vi "Rename_Folder_of_VIs.vi"() -> ()   [LabVIEW 2009]
uses:
  <userlib>/_OpenG.lib/file/file.llb/Build Path - File Names Array__ogtk.vi
  <userlib>/_OpenG.lib/file/file.llb/Strip Path Extension - String__ogtk.vi
  <userlib>/_OpenG.lib/file/file.llb/Strip Path Extension - Path__ogtk.vi
  <userlib>/_OpenG.lib/comparison/comparison.llb/I32 Changed__ogtk.vi
  <userlib>/_OpenG.lib/file/file.llb/Valid Path - Traditional__ogtk.vi
  <userlib>/_OpenG.lib/comparison/comparison.llb/Variant Changed__ogtk.vi
  <userlib>/_OpenG.lib/file/file.llb/Strip Path Extension - 1D Array of Strings__ogtk.vi
panel:
  in  "Swap":bool
  in  "About":bool
  in  "Source Folder":path caption="Folder"
  in  "Folder or LLB":enum32{"Folder", "LLB"}(radio)
  out "Total Progress":u8(slide) scale=0.0..100.0
  out "Progress":u8(slide) scale=0.0..100.0
  in  "Prefix or Suffix":enum32{"Prefix", "Suffix"}(radio)
  in  "Exit Button":bool
  in  "Rename Button":bool
  in  "Recursive":bool
  in  "New Prefix":string caption="New Prefix (\"\": remove existing prefix)"
  in  "Existing Prefix":string caption="Existing Prefix (\"\": prepend new prefix)"
  # "Options"
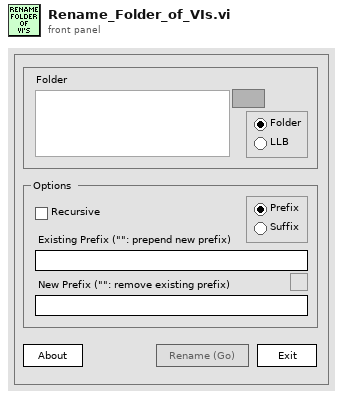
[diagram p1: front panel]
types:
  T1 = cluster{"Version":string, "Build Number":u32, "Build Date/Time":dbl}
  T2 = enum8{"Enabled", "Disabled", "Disabled and Grayed Out"}
  T3 = enum32{"invalid VI type", "Standard VI", "Control VI", "Global VI", "Polymorphic VI", "Configuration VI"}
  T4 = enum32{"invalid VI type", "Standard VI", "Control VI", "Global VI", "Polymorphic VI", "Configuration VI", "SubSystem", "Facade VI", "Method VI", "Statechart Diagram VI"}
  T5 = cluster{"Prompt":string, "Match Pattern":string, "Mode":u32, "Start Path":path}
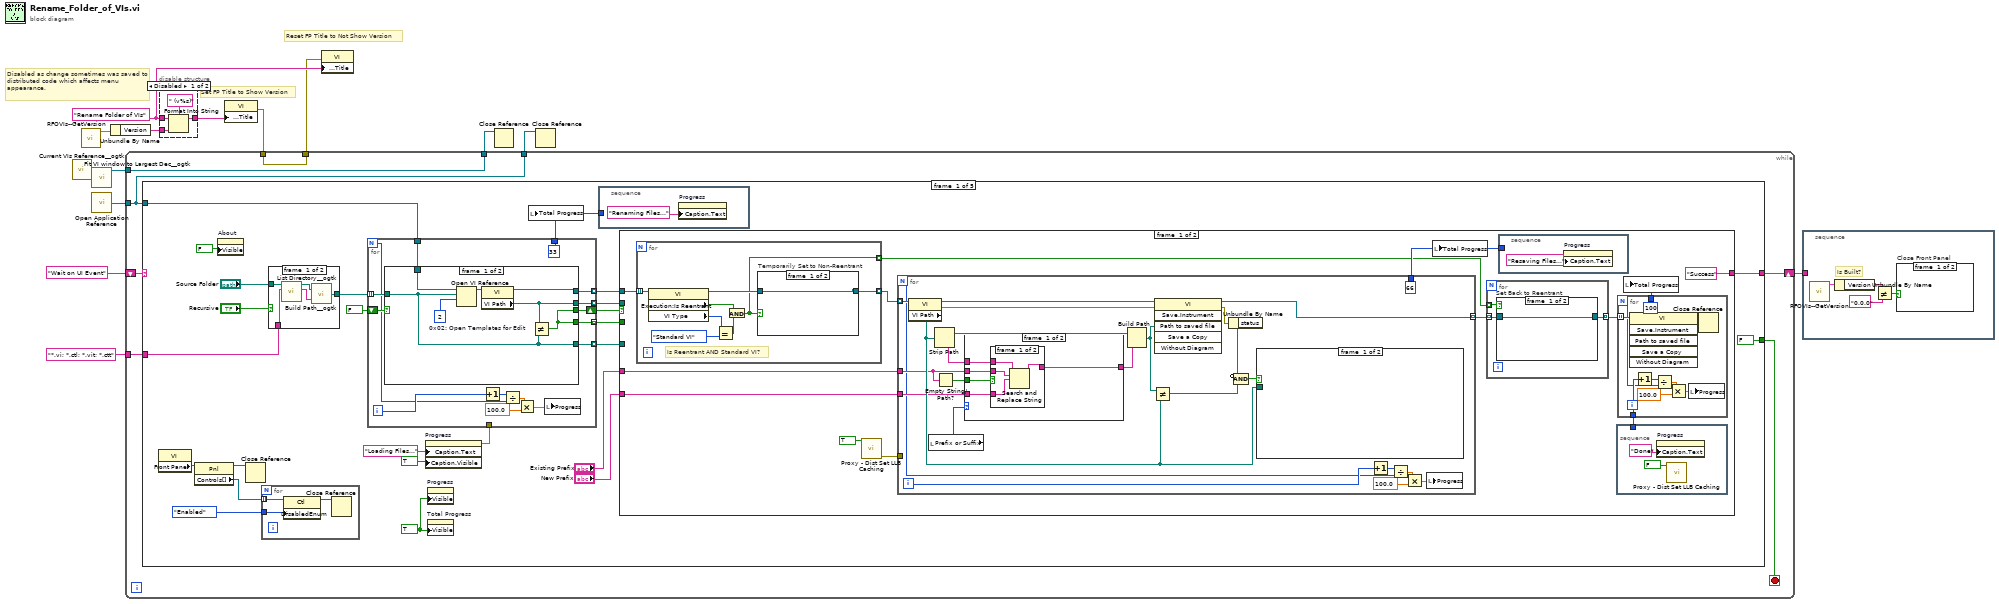
[diagram p0: block diagram]
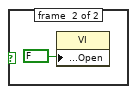
[diagram p3: hidden frame]
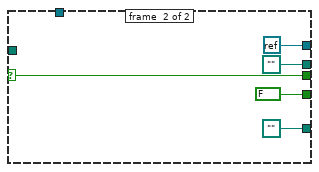
[diagram p4: hidden frame]
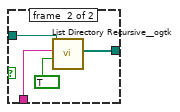
[diagram p5: hidden frame]
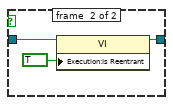
[diagram p6: hidden frame]
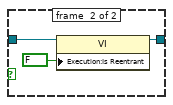
[diagram p7: hidden frame]
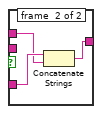
[diagram p8: hidden frame]
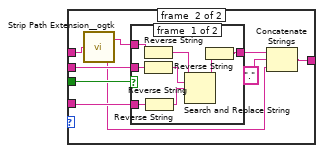
[diagram p9: hidden frame]
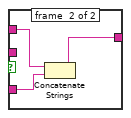
[diagram p10: hidden frame]
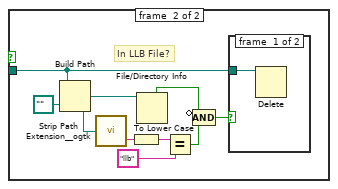
[diagram p11: hidden frame]
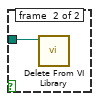
[diagram p12: hidden frame]
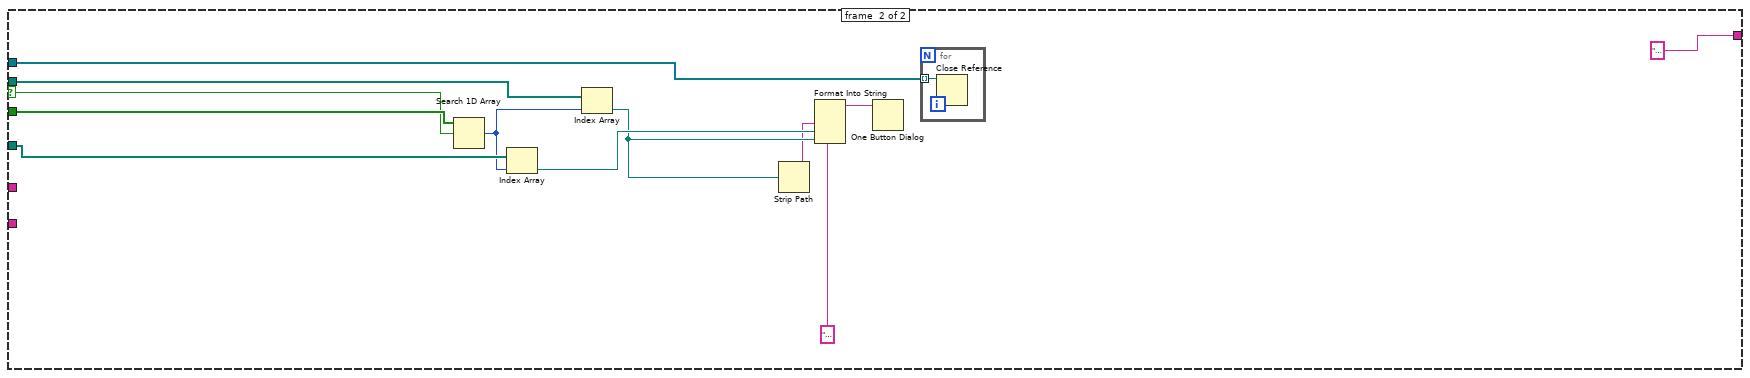
[diagram p13: hidden frame]
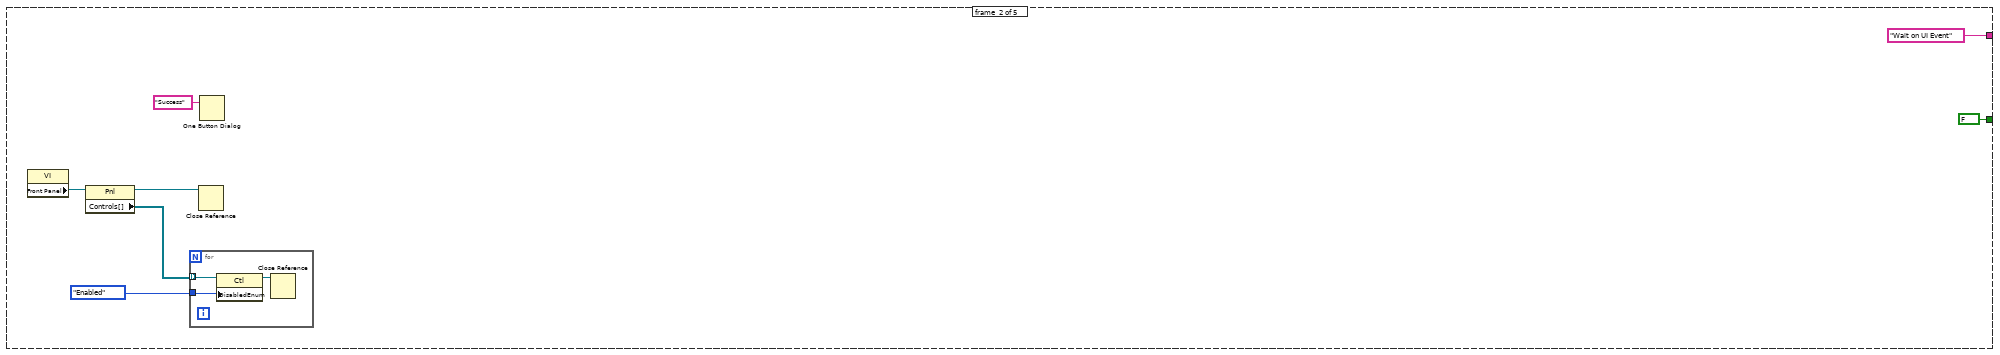
[diagram p14: hidden frame]
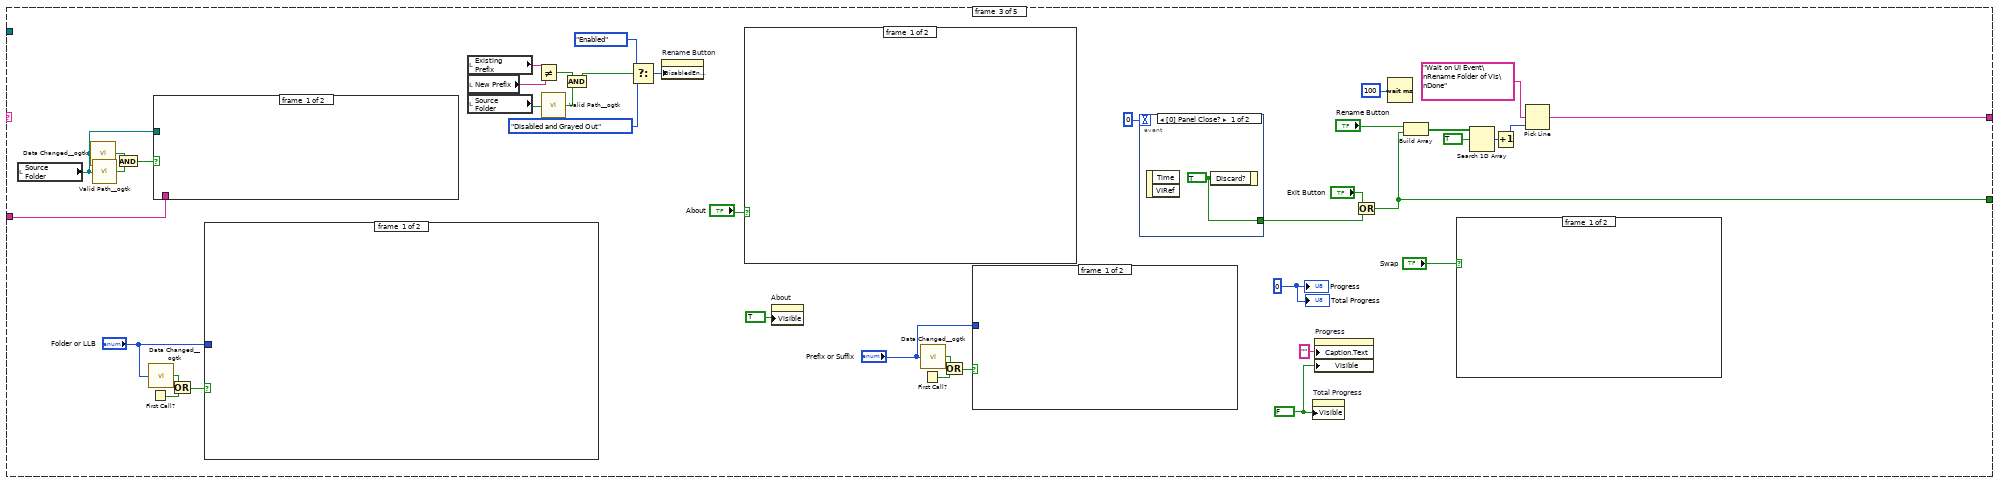
[diagram p15: hidden frame]
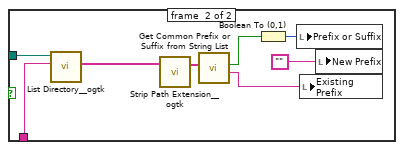
[diagram p16: hidden frame]
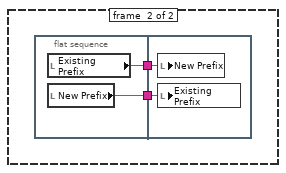
[diagram p17: hidden frame]
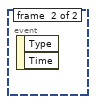
[diagram p18: hidden frame]
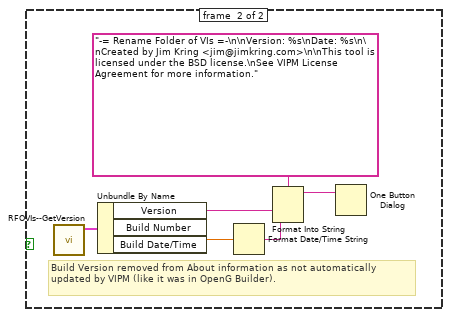
[diagram p19: hidden frame]
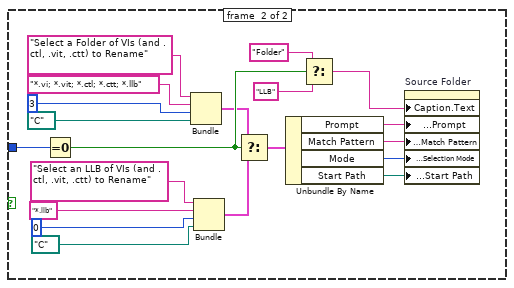
[diagram p20: hidden frame]
diagram:
  w8 = "Rename Folder of VIs" ("format string")
  # "Disabled as change sometimes was saved to distributed code which affects menu appearance."
  # "Set FP Title to Show Version"
  # "Reset FP Title to Not Show Version"
  n1 = call <userlib>:"Current VIs Reference__ogtk.vi"() -> ("Current VI's reference"=w13:refnum<vi>)  [unwired: 5 in]
  n2 = call "RFOVIs--GetVersion.vi"() -> ("Version Info"=w11:T1)  [unwired: 10 in, 1 out]
  n3 = call <userlib>:"Fit VI window to Largest Dec__ogtk.vi"("VI Ref (calling VI)"=w13) -> ("dup VI Ref"=w12:refnum<vi>)  [unwired: 5 in, 1 out]
  n4 = call "Open Application Reference.vi"() -> ("application reference"=w5:refnum<vi>)
  n5 = Unbundle By Name(w11) -> ("Version"=w10:string)
  n6 = disable-structure shown="Disabled" {
    disable-tunnel: w10 -> [w18 _]
    disable-tunnel: [w16 w19] -> w9
    disable-tunnel: w8 -> [w15 w19]
    frame #0 {
      n7 = Format Into String(format string=" (v%s)", initial string=w15, w18) -> (resulting string=w16:string)  [unwired: 1 in, 1 out]
    }
    frame #1 {
    }
  }
  n8 = property class="VI"("Front Panel Window:Title"=w9) -> (error out=w2:errorcluster)  [unwired: 2 in, 1 out]
  n9 = while {
    tunnel: w12 -> [w22]
    shift-left: "Wait on UI Event" -> [w26]
    shift-right: [w24] -> w7
    tunnel: [w23] -> w1
    tunnel: w2 -> [w23]
    tunnel: [w22] -> w6
    tunnel: w5 -> [w21]
    tunnel: [w21] -> w4
    tunnel: "*.vi; *.ctl; *.vit; *.ctt" ("pattern") -> [w20]
    stop <- w25 stop-if-true
    n10 = case shown="\"Wait on UI Event\"" w26 {
      selector: w26 -> [_ _ _ w316 _]
      tunnel: [FALSE ("Cancel") FALSE ("Cancel") w243 FALSE ("Cancel") TRUE ("Cancel")] -> w25
      tunnel: [w27 "Wait on UI Event" ("pattern") w253 "Wait on UI Event" ("pattern") "" ("pattern")] -> w24
      tunnel: w21 -> [w33 _ _ _ _]
      tunnel: w20 -> [w29 _ w230 _ _]
      frame #0 {
        w35 = TRUE ("Visible")
        n11 = property class="VI"() -> ("Front Panel"=w40:refnum<vi>)  [unwired: 2 in, 2 out]
        n12 = property class="Pnl"(reference=w40) -> (reference out=w38:refnum<vi>, "Controls[]"=w39:refnum<vi>[])  [unwired: 1 in, 1 out]
        n13 = property on="About" class="Boolean"("Visible"=FALSE) -> ()  [unwired: 2 in, 2 out]
        n14 = Close Reference(reference=w38) -> ()  [unwired: 1 in, 1 out]
        n15 = for {
          tunnel: w39 -> [w55] mode=indexing
          tunnel: T2."Enabled" ("Disabled") -> [w53]
          n16 = property on="Property Node" class="Ctl"(reference=w55, "DisabledEnum"=w53) -> (reference out=w54:refnum<vi>)  [unwired: 1 in, 1 out]
          n17 = Close Reference(reference=w54) -> ()  [unwired: 1 in, 1 out]
        }
        n18 = case shown="False" "Recursive" {
          tunnel: "Source Folder" -> [w87 w91]
          tunnel: [w83 w90] -> w44
          tunnel: w29 -> [w86 w89]
          frame #0 {
            n19 = call <userlib>:"List Directory__ogtk.vi"("pattern"=w86, "directory path"=w87) -> ("file names"=w84:string[], "dup directory path"=w85:path)  [unwired: 2 in, 2 out]
            n20 = call-poly <userlib>:"Build Path__ogtk.vi"("name or relative path"=w84, "base path"=w85) -> ("appended path"=w83:path[])
          }
          frame #1 {
            n21 = call <userlib>:"List Directory Recursive__ogtk.vi"("Treat llb files as directories? (FALSE)"=TRUE, "pattern"=w89, "Path"=w91) -> ("file paths"=w90:path[])  [unwired: 5 in, 3 out]
          }
        }
        n22 = property on="Progress" class="Slide (strict)"("Caption.Text"="Loading Files...", "Caption.Visible"=TRUE) -> (error out=w31:errorcluster)  [unwired: 2 in, 1 out]
        n23 = for {
          N -> [w58]
          tunnel: w44 -> [w69] mode=indexing
          tunnel: [w70] -> w45 mode=indexing
          shift-right: [w68] -> w48
          shift-left: FALSE -> [w67]
          tunnel: [w66] -> w49 mode=indexing
          tunnel: [w65] -> w50 mode=indexing
          tunnel: [w64] -> w51 mode=indexing
          tunnel: [u8 33 ("Total Progress")] -> w36
          tunnel: w33 -> [w56]
          tunnel: w31 -> [_]
          i -> [w59]
          n24 = case shown="False" w67 {
            selector: w67 -> [_ w82]
            tunnel: [w76 refnum<k0> refnum] -> w70
            tunnel: w69 -> [w73 _]
            tunnel: [w75 w82] -> w68
            tunnel: [w75 FALSE] -> w66
            tunnel: [w73 path ""] -> w65
            tunnel: [w74 path "" ("Path")] -> w64
            tunnel: w56 -> [w71 _]
            frame #0 {
              w72 = 2  # 0x02: Open Templates for Edit
              n25 = Open VI Reference(application reference (local)=w71, vi path=w73, options=w72) -> (vi reference=w77:refnum<vi>)  [unwired: 3 in, 1 out]
              n26 = property class="VI"(reference=w77) -> (reference out=w76:refnum<vi>, "VI Path"=w74:path)  [unwired: 1 in, 1 out]
              n27 = Not Equal?(x=w74, y=w73) -> (x != y?=w75:bool)
            }
            frame #1 {
            }
          }
          n28 = Increment(x=w59) -> (x+1=w60:i32)
          n29 = Divide(x=w60, y=w58) -> (x/y=w62:dbl)
          n30 = Multiply(x=w62, y=100.0) -> (x*y=w63:dbl)
          n31 = local write "Progress"(w63) -> ()
        }
        n32 = property on="Progress" class="Slide (strict)"("Visible"=w35) -> ()  [unwired: 2 in, 2 out]
        n33 = property on="Total Progress" class="Slide (strict)"("Visible"=w35) -> ()  [unwired: 2 in, 2 out]
        n34 = local write "Total Progress"(w36) -> ()
        n35 = stacked-sequence {
          tunnel: w36 -> [_]
          frame #0 {
            n36 = property on="Progress" class="Slide (strict)"("Caption.Text"="Renaming Files...") -> ()  [unwired: 2 in, 2 out]
          }
        }
        n37 = case shown="False" w48 {
          selector: w48 -> [_ w213]
          tunnel: "Existing Prefix" -> [w104 _]
          tunnel: "New Prefix" -> [w103 _]
          tunnel: w45 -> [w98 w212]
          tunnel: w49 -> [_ w214]
          tunnel: w50 -> [_ w211]
          tunnel: w51 -> [_ w210]
          tunnel: ["Success" ("pattern") "Wait on UI Event" ("pattern")] -> w27
          frame #0 {
            n38 = for {
              tunnel: w98 -> [w119] mode=indexing
              tunnel: [w113] -> w94 mode=indexing
              tunnel: [w112] -> w97 mode=indexing
              # "Is Reentrant AND Standard VI?"
              n39 = property class="VI"(reference=w119) -> (reference out=w114:refnum<vi>, "Execution:Is Reentrant"=w115:bool, "VI Type"=w117:T4)  [unwired: 1 in, 1 out]
              n40 = Equal?(x=w117, y=T3."Standard VI" ("VI Type")) -> (x = y?=w116:bool)
              n41 = And(x=w115, y=w116) -> (x .and. y?=w113:bool)
              n42 = case "Temporarily Set to Non-Reentrant" shown="True" w113 {
                tunnel: w114 -> [w120 w123]
                tunnel: [w120 w121] -> w112
                frame #0 {
                }
                frame #1 {
                  n43 = property class="VI"(reference=w123, "Execution:Is Reentrant"=FALSE) -> (reference out=w121:refnum<vi>)  [unwired: 1 in, 1 out]
                }
              }
            }
            n44 = call "Proxy - Dist Set LLB Caching.vi"("enable?"=TRUE) -> ("error out"=w92:errorcluster)  [unwired: 10 in]
            n45 = for {
              N -> [w138]
              tunnel: w104 -> [w149]
              tunnel: w103 -> [w150]
              tunnel: w97 -> [w147] mode=indexing
              tunnel: [w145] -> w96 mode=indexing
              tunnel: [u8 66 ("Total Progress")] -> w101
              tunnel: w92 -> [_]
              i -> [w139]
              n46 = property class="VI"(reference=w147) -> (reference out=w156:refnum<vi>, error out=w155:errorcluster, "VI Path"=w151:path)  [unwired: 1 in]
              n47 = local read "Prefix or Suffix"() -> (w144:enum32{"Prefix", "Suffix"})
              n48 = Strip Path(path=w151) -> (stripped path=w159:path, name=w158:string)
              n49 = Empty String/Path?(string/path=w149) -> (empty?=w148:bool)
              n50 = case shown="\"Prefix\", Default" w144 {
                tunnel: w158 -> [w164 w180]
                tunnel: [w163 w172] -> w157
                tunnel: w150 -> [w162 w177]
                tunnel: w149 -> [w161 w176]
                tunnel: w148 -> [w160 w179]
                frame #0 {
                  n51 = case shown="True" w160 {
                    tunnel: w164 -> [w168 w170]
                    tunnel: [w167 w169] -> w163
                    tunnel: w162 -> [w166 w171]
                    tunnel: w161 -> [w165 _]
                    frame #0 {
                      n52 = Search and Replace String(input string=w168, search string=w165, replace string=w166) -> (result string=w167:string)  [unwired: 5 in, 3 out]
                    }
                    frame #1 {
                      n53 = Concatenate Strings(w171, w170) -> (w169:string)
                    }
                  }
                }
                frame #1 {
                  n54 = call-poly <userlib>:"Strip Path Extension__ogtk.vi"("path"=w180) -> ("root"=w178:string, "extension"=w173:string)
                  n55 = case shown="False" w179 {
                    tunnel: [w184 w191] -> w174
                    tunnel: w177 -> [w187 w189]
                    tunnel: w178 -> [w181 w190]
                    tunnel: w176 -> [w188 _]
                    frame #0 {
                      n56 = Reverse String(1:w181) -> (0:w182:string)
                      n57 = Reverse String(1:w188) -> (0:w186:string)
                      n58 = Reverse String(1:w187) -> (0:w185:string)
                      n59 = Search and Replace String(input string=w182, search string=w186, replace string=w185) -> (result string=w183:string)  [unwired: 5 in, 3 out]
                      n60 = Reverse String(1:w183) -> (0:w184:string)
                    }
                    frame #1 {
                      n61 = Concatenate Strings(w190, w189) -> (w191:string)
                    }
                  }
                  n62 = Concatenate Strings(w174, "." ("Substring"), w173) -> (w172:string)
                }
              }
              n63 = Build Path(base path=w159, name or relative path=w157) -> (appended path=w154:path)
              n64 = Not Equal?(x=w154, y=w151) -> (x != y?=w153:bool)
              n65 = invoke class="VI" method="Save.Instrument"(reference=w156, error in=w155, "Path to saved file"=w154) -> (reference out=w145:refnum<vi>, error out=w146:errorcluster)  [unwired: 3 in, 4 out]
              n66 = Unbundle By Name(w146) -> ("status"=w136:bool)
              n67 = Compound Arithmetic op=AND(invert w136, w153) -> (w152:bool)
              n68 = case shown="True" w152 {
                tunnel: w151 -> [_ w192]
                frame #0 {
                }
                frame #1 {
                  # "In LLB File?"
                  n69 = Build Path(base path=w192, name or relative path=path ".." ("base path")) -> (appended path=w199:path)
                  n70 = call-poly <userlib>:"Strip Path Extension__ogtk.vi"("path"=w199) -> ("extension"=w198:string)  [unwired: 1 out]
                  n71 = To Lower Case(string=w198) -> (all lower case string=w197:string)
                  n72 = File/Directory Info(path=w199) -> (directory=w195:bool)  [unwired: 1 in, 6 out]
                  n73 = Equal?(x=w197, y="llb" ("all lower case string")) -> (x = y?=w194:bool)
                  n74 = Compound Arithmetic op=AND(invert w195, w194) -> (w193:bool)
                  n75 = case shown="True" w193 {
                    tunnel: w192 -> [w201 w202]
                    frame #0 {
                      n76 = Delete(path (use dialog)=w201) -> ()  [unwired: 4 in, 3 out]
                    }
                    frame #1 {
                      n77 = call <vilib>:"Delete From VI Library.vi"("path"=w202) -> ()  [unwired: 10 in, 1 out]
                    }
                  }
                }
              }
              n78 = Increment(x=w139) -> (x+1=w140:i32)
              n79 = Divide(x=w140, y=w138) -> (x/y=w142:dbl)
              n80 = Multiply(x=w142, y=100.0) -> (x*y=w143:dbl)
              n81 = local write "Progress"(w143) -> ()
            }
            n82 = local write "Total Progress"(w101) -> ()
            n83 = for {
              tunnel: [w107] -> w95 mode=indexing
              tunnel: w96 -> [w106] mode=indexing
              tunnel: w94 -> [w105] mode=indexing
              n84 = case "Set Back to Reentrant" shown="True" w105 {
                tunnel: w106 -> [w108 w111]
                tunnel: [w108 w109] -> w107
                frame #0 {
                }
                frame #1 {
                  n85 = property class="VI"(reference=w111, "Execution:Is Reentrant"=TRUE) -> (reference out=w109:refnum<vi>)  [unwired: 1 in, 1 out]
                }
              }
            }
            n86 = stacked-sequence {
              tunnel: w101 -> [_]
              frame #0 {
                n87 = property on="Progress" class="Slide (strict)"("Caption.Text"="Resaving Files...") -> ()  [unwired: 2 in, 2 out]
              }
            }
            n88 = for {
              N -> [w128]
              tunnel: w95 -> [w135] mode=indexing
              tunnel: [u8 100 ("Total Progress")] -> w100
              tunnel: [w129] -> w99
              i -> [w129]
              n89 = invoke class="VI" method="Save.Instrument"(reference=w135) -> (reference out=w134:refnum<vi>)  [unwired: 5 in, 5 out]
              n90 = Increment(x=w129) -> (x+1=w130:i32)
              n91 = Divide(x=w130, y=w128) -> (x/y=w132:dbl)
              n92 = Multiply(x=w132, y=100.0) -> (x*y=w133:dbl)
              n93 = local write "Progress"(w133) -> ()
              n94 = Close Reference(reference=w134) -> ()  [unwired: 1 in, 1 out]
            }
            n95 = stacked-sequence {
              tunnel: w99 -> [_]
              frame #0 {
                n96 = property on="Progress" class="Slide (strict)"("Caption.Text"="Done") -> ()  [unwired: 2 in, 2 out]
                n97 = call "Proxy - Dist Set LLB Caching.vi"("enable?"=FALSE) -> ()  [unwired: 10 in, 1 out]
              }
            }
            n98 = local write "Total Progress"(w100) -> ()
          }
          frame #1 {
            n99 = Search 1D Array(1D array=w214, element=w213) -> (index of element=w209:i32)  [unwired: 1 in]
            n100 = Index Array(array=w211, index=w209) -> (element=w208:path)
            n101 = Index Array(array=w210, index=w209) -> (element=w207:path)
            n102 = Strip Path(path=w207) -> (name=w206:string)  [unwired: 1 out]
            n103 = Format Into String(format string="Cannot rename folder. \"%s\" expected in the following location:\n\n%s\n\nfound already in memory at:\n\n%s\n\nNo VIs renamed.", w206, w208, w207) -> (resulting string=w205:string)  [unwired: 2 in, 1 out]
            n104 = One Button Dialog(message=w205) -> ()  [unwired: 1 in, 1 out]
            n105 = for {
              tunnel: w212 -> [w215] mode=indexing
              n106 = Close Reference(reference=w215) -> ()  [unwired: 1 in, 1 out]
            }
          }
        }
      }
      frame #1 {
        n107 = property class="VI"() -> ("Front Panel"=w220:refnum<vi>)  [unwired: 2 in, 2 out]
        n108 = property class="Pnl"(reference=w220) -> (reference out=w218:refnum<vi>, "Controls[]"=w219:refnum<vi>[])  [unwired: 1 in, 1 out]
        n109 = for {
          tunnel: w219 -> [w225] mode=indexing
          tunnel: T2."Enabled" ("Disabled") -> [w223]
          n110 = property on="Property Node" class="Ctl"(reference=w225, "DisabledEnum"=w223) -> (reference out=w224:refnum<vi>)  [unwired: 1 in, 1 out]
          n111 = Close Reference(reference=w224) -> ()  [unwired: 1 in, 1 out]
        }
        n112 = Close Reference(reference=w218) -> ()  [unwired: 1 in, 1 out]
        n113 = One Button Dialog(message="Success") -> ()  [unwired: 1 in, 1 out]
      }
      frame #2 {
        w251 = FALSE ("Visible")
        w252 = u8 0 ("Progress")
        n114 = local read "Source Folder"() -> (w229:path)
        n115 = call-poly <userlib>:"Data Changed__ogtk.vi"("Variant"=w229) -> ("Changed"=w233:bool)
        n116 = call-poly <userlib>:"Valid Path__ogtk.vi"("path"=w229) -> ("valid"=w232:bool)
        n117 = And(x=w233, y=w232) -> (x .and. y?=w231:bool)
        n118 = First Call?() -> (First Call?: T/F=w248:bool)
        n119 = call-poly <userlib>:"Data Changed__ogtk.vi"("I32"="Folder or LLB") -> ("Changed"=w247:bool)
        n120 = case shown="True" w231 {
          tunnel: w229 -> [_ w273]
          tunnel: w230 -> [_ w272]
          frame #0 {
          }
          frame #1 {
            n121 = call <userlib>:"List Directory__ogtk.vi"("pattern"=w272, "directory path"=w273) -> ("file names"=w271:string[])  [unwired: 2 in, 3 out]
            n122 = call-poly <userlib>:"Strip Path Extension__ogtk.vi"("paths"=w271) -> ("roots"=w270:string[])  [unwired: 1 out]
            n123 = call "Get Common Prefix or Suffix from String List.vi"("Strings"=w270) -> ("Common Part"=w268:string, "Suffix? (F: Prefix)"=w267:bool)  [unwired: 9 in]
            n124 = Boolean To (0,1)(Boolean=w267) -> (0, 1=w266:i16)
            n125 = local write "Prefix or Suffix"(w266) -> ()
            n126 = local write "Existing Prefix"(w268) -> ()
            n127 = local write "New Prefix"("") -> ()
          }
        }
        n128 = Or(x=w247, y=w248) -> (x .or. y?=w249:bool)
        n129 = case shown="True" w249 {
          tunnel: "Folder or LLB" -> [_ w305]
          frame #0 {
          }
          frame #1 {
            n130 = Equal To 0?(x=w305) -> (x = 0?=w304:bool)
            n131 = Bundle("Prompt"="Select a Folder of VIs (and .ctl, .vit, .ctt) to Rename", "Match Pattern"="*.vi; *.vit; *.ctl; *.ctt; *.llb", "Mode"=u32 3, "Start Path"=path "C:/") -> (w293:T5)  [unwired: 1 in]
            n132 = Bundle("Prompt"="Select an LLB of VIs (and .ctl, .vit, .ctt) to Rename", "Match Pattern"="*.llb", "Mode"=u32 0, "Start Path"=path "C:/") -> (w294:T5)  [unwired: 1 in]
            n133 = Select(t=w293, s=w304, f=w294) -> (s? t:f=w292:T5)
            n134 = Unbundle By Name(w292) -> ("Prompt"=w291:string, "Match Pattern"=w290:string, "Mode"=w289:u32, "Start Path"=w288:path)
            n135 = Select(t="Folder", s=w304, f="LLB") -> (s? t:f=w287:string)
            n136 = property on="Source Folder" class="Path"("Caption.Text"=w287, "Browse Options:Prompt"=w291, "Browse Options:Match Pattern"=w290, "Browse Options:Selection Mode"=w289, "Browse Options:Start Path"=w288) -> ()  [unwired: 2 in, 2 out]
          }
        }
        n137 = local read "Existing Prefix"() -> (w240:string)
        n138 = local read "New Prefix"() -> (w239:string)
        n139 = local read "Source Folder"() -> (w238:path)
        n140 = Not Equal?(x=w240, y=w239) -> (x != y?=w237:bool)
        n141 = call-poly <userlib>:"Valid Path__ogtk.vi"("path"=w238) -> ("valid"=w236:bool)
        n142 = And(x=w237, y=w236) -> (x .and. y?=w235:bool)
        n143 = Select(t=T2."Enabled" ("Disabled"), s=w235, f=T2."Disabled and Grayed Out" ("Disabled")) -> (s? t:f=w227:T2)
        n144 = property on="Rename Button" class="Boolean"("DisabledEnum"=w227) -> ()  [unwired: 2 in, 2 out]
        n145 = case shown="True" "About" {
          frame #0 {
          }
          frame #1 {
            # "Build Version removed from About information as not automatically updated by VIPM (like it was in OpenG Builder)."
            n146 = call "RFOVIs--GetVersion.vi"() -> ("Version Info"=w285:T1)  [unwired: 10 in, 1 out]
            n147 = Unbundle By Name(w285) -> ("Version"=w284:string, "Build Date/Time"=w282:dbl)  [unwired: 1 out]
            n148 = Format Date/Time String(seconds (now)=w282) -> (date/time string=w281:string)  [unwired: 2 in]
            n149 = Format Into String(format string="-= Rename Folder of VIs =-\n\nVersion: %s\nDate: %s\n\nCreated by Jim Kring <jim@jimkring.com>\n\nThis tool is licensed under the BSD license.\nSee VIPM License Agreement for more information." ("pattern"), w284, w281) -> (resulting string=w283:string)  [unwired: 2 in, 1 out]
            n150 = One Button Dialog(message=w283) -> ()  [unwired: 1 in, 1 out]
          }
        }
        n151 = property on="About" class="Boolean"("Visible"=TRUE) -> ()  [unwired: 2 in, 2 out]
        n152 = First Call?() -> (First Call?: T/F=w263:bool)
        n153 = call-poly <userlib>:"Data Changed__ogtk.vi"("I32"="Prefix or Suffix") -> ("Changed"=w264:bool)
        n154 = Or(x=w264, y=w263) -> (x .or. y?=w262:bool)
        n155 = case shown="True" w262 {
          tunnel: "Prefix or Suffix" -> [_ w311]
          frame #0 {
          }
          frame #1 {
            n156 = Pick Line(multi-line string="Existing Prefix (\"\": prepend new prefix)\nExisting Suffix (\"\": apend new prefix)", line index=w311) -> (output string=w308:string)  [unwired: 1 in]
            n157 = Pick Line(multi-line string="New Prefix (\"\": remove existing prefix)\nNew Suffix (\"\": remove existing suffix)", line index=w311) -> (output string=w307:string)  [unwired: 1 in]
            n158 = property on="Existing Prefix" class="String"("Caption.Text"=w308) -> ()  [unwired: 2 in, 2 out]
            n159 = property on="New Prefix" class="String"("Caption.Text"=w307) -> ()  [unwired: 2 in, 2 out]
          }
        }
        n160 = event shown="[0] Panel Close?" {
          selector: _ -> [_ _]
          dyn-events: _ -> [_ _]
          timeout: 0 -> [_ _]
          tunnel: [w280 _] -> w244
          event #0 {
            w280 = TRUE ("Discard?")
            n161 = event-data() -> ()  [unwired: 1 in, 2 out]
            n162 = event-data("Discard?"=w280) -> ()  [unwired: 1 in, 1 out]
          }
          event #1 {
            n163 = event-data() -> ()  [unwired: 1 in, 2 out]
          }
        }
        n164 = property on="Total Progress" class="Slide (strict)"("Visible"=w251) -> ()  [unwired: 2 in, 2 out]
        n165 = property on="Progress" class="Slide (strict)"("Caption.Text"="", "Visible"=w251) -> ()  [unwired: 2 in, 2 out]
        n166 = Or(x="Exit Button", y=w244) -> (x .or. y?=w243:bool)
        n167 = Wait (ms)(milliseconds to wait=u32 100) -> ()  [unwired: 1 out]
        n168 = Build Array("Rename Button", w243) -> (w259:bool[])
        n169 = case shown="True" "Swap" {
          frame #0 {
          }
          frame #1 {
            n170 = flat-sequence {
              tunnel: [w277] -> w275
              tunnel: [w276] -> w274
              tunnel: w275 -> [w279]
              tunnel: w274 -> [w278]
              frame #0 {
                n171 = local read "Existing Prefix"() -> (w277:string)
                n172 = local read "New Prefix"() -> (w276:string)
              }
              frame #1 {
                n173 = local write "New Prefix"(w279) -> ()
                n174 = local write "Existing Prefix"(w278) -> ()
              }
            }
          }
        }
        n175 = Search 1D Array(1D array=w259, element=TRUE) -> (index of element=w257:i32)  [unwired: 1 in]
        n176 = Increment(x=w257) -> (x+1=w256:i32)
        n177 = Pick Line(multi-line string="Wait on UI Event\nRename Folder of VIs\nDone" ("pattern"), line index=w256) -> (output string=w253:string)  [unwired: 1 in]
        "Total Progress" <- w252
        "Progress" <- w252
      }
      frame #3 {
        n178 = Format Into String(format string="Error Undefined Software State \"%s\"", w316) -> (resulting string=w313:string)  [unwired: 2 in, 1 out]
        n179 = One Button Dialog(message=w313) -> ()  [unwired: 1 in, 1 out]
      }
      frame #4 {
      }
    }
  }
  n180 = property class="VI"(error in=w1, "Front Panel Window:Title"=w8) -> ()  [unwired: 1 in, 2 out]
  n181 = Close Reference(reference=w6) -> ()  [unwired: 1 in, 1 out]
  n182 = Close Reference(reference=w4) -> ()  [unwired: 1 in, 1 out]
  n183 = stacked-sequence {
    tunnel: w7 -> [_]
    frame #0 {
      # "Is Built?"
      n184 = call "RFOVIs--GetVersion.vi"() -> ("Version Info"=w322:T1)  [unwired: 10 in, 1 out]
      n185 = Unbundle By Name(w322) -> ("Version"=w321:string)
      n186 = Not Equal?(x=w321, y="0.0.0" ("Version")) -> (x != y?=w319:bool)
      n187 = case "Close Front Panel" shown="True" w319 {
        frame #0 {
        }
        frame #1 {
          n188 = property class="VI"("Front Panel Window:Open"=FALSE) -> ()  [unwired: 2 in, 2 out]
        }
      }
    }
  }
